vi "splice_intelligent_normalized_2.0.vi"(8 "xmax":dbl, 9 "xmin":dbl, 10 "X":dbl[](array[numeric]), 11 "Y":dbl[](array[numeric])) -> (0 "Splice indices":i32[](array[numeric]), 1 "Extrema type (T=max, F=min)":bool[](array[boolean]), 2 "X splices":cluster{dbl[]}[](array[cluster]), 3 "Y splices":cluster{dbl[]}[](array[cluster]), 4 "Extrema (indices)":i32[](array[numeric]))   [LabVIEW 2019]
uses:
  <vilib>/ptbypt/NI_PtbyPt.lvlib
panel:
  out "XY Graph":cluster{"X":dbl[], "Y":dbl[]}(graph)
  out "Array":cluster{"XY Graph":cluster{dbl[], dbl[]}}[](array[cluster])
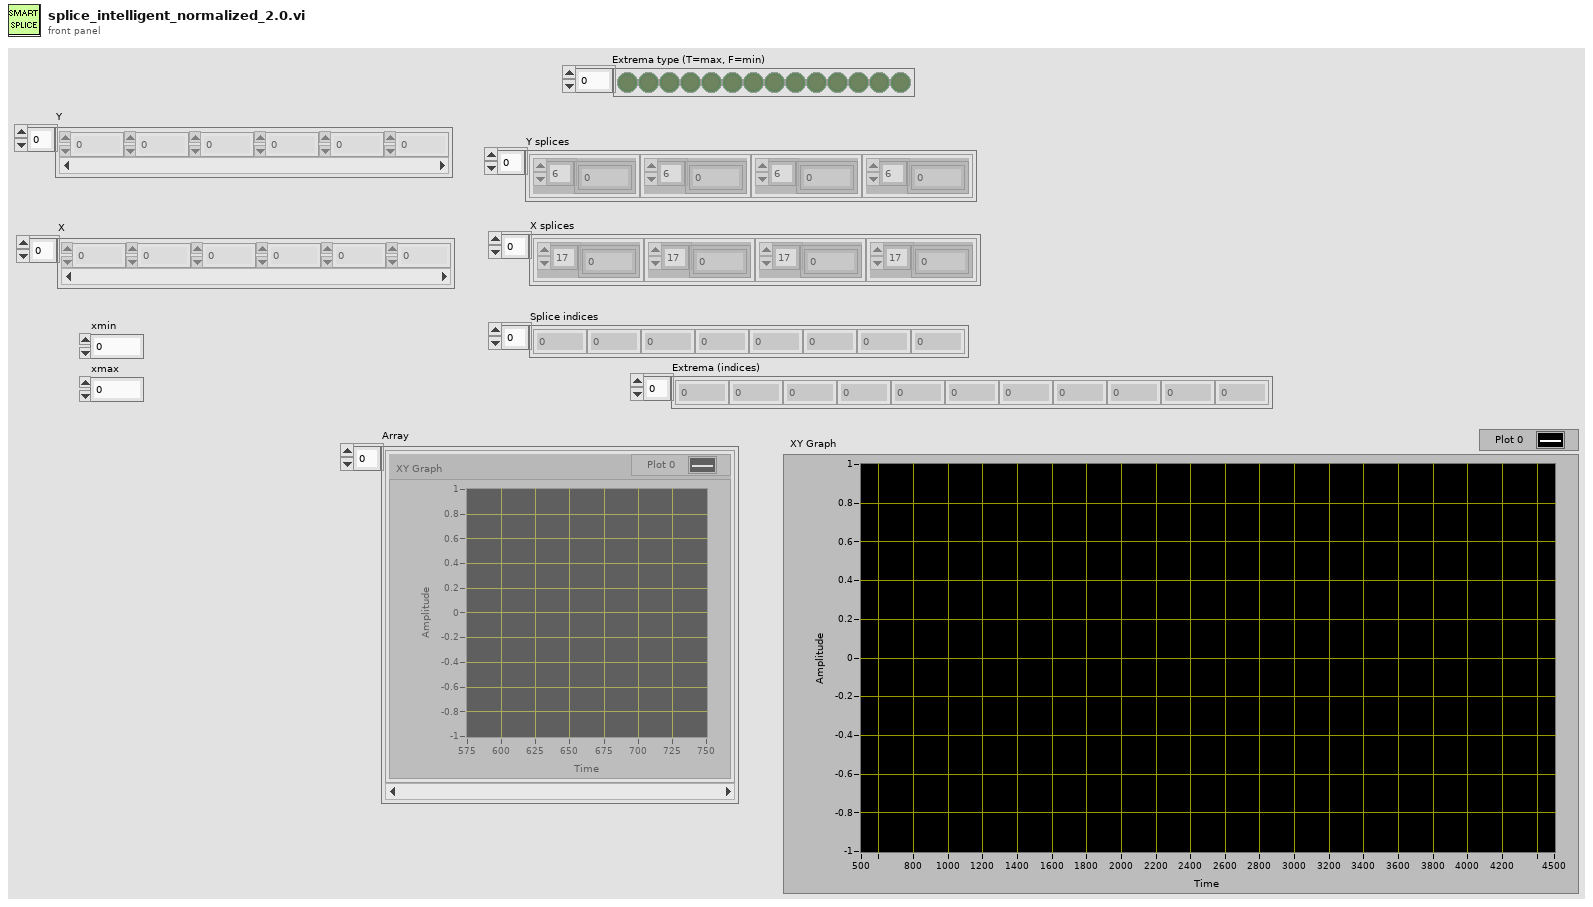
[diagram p1: front panel]
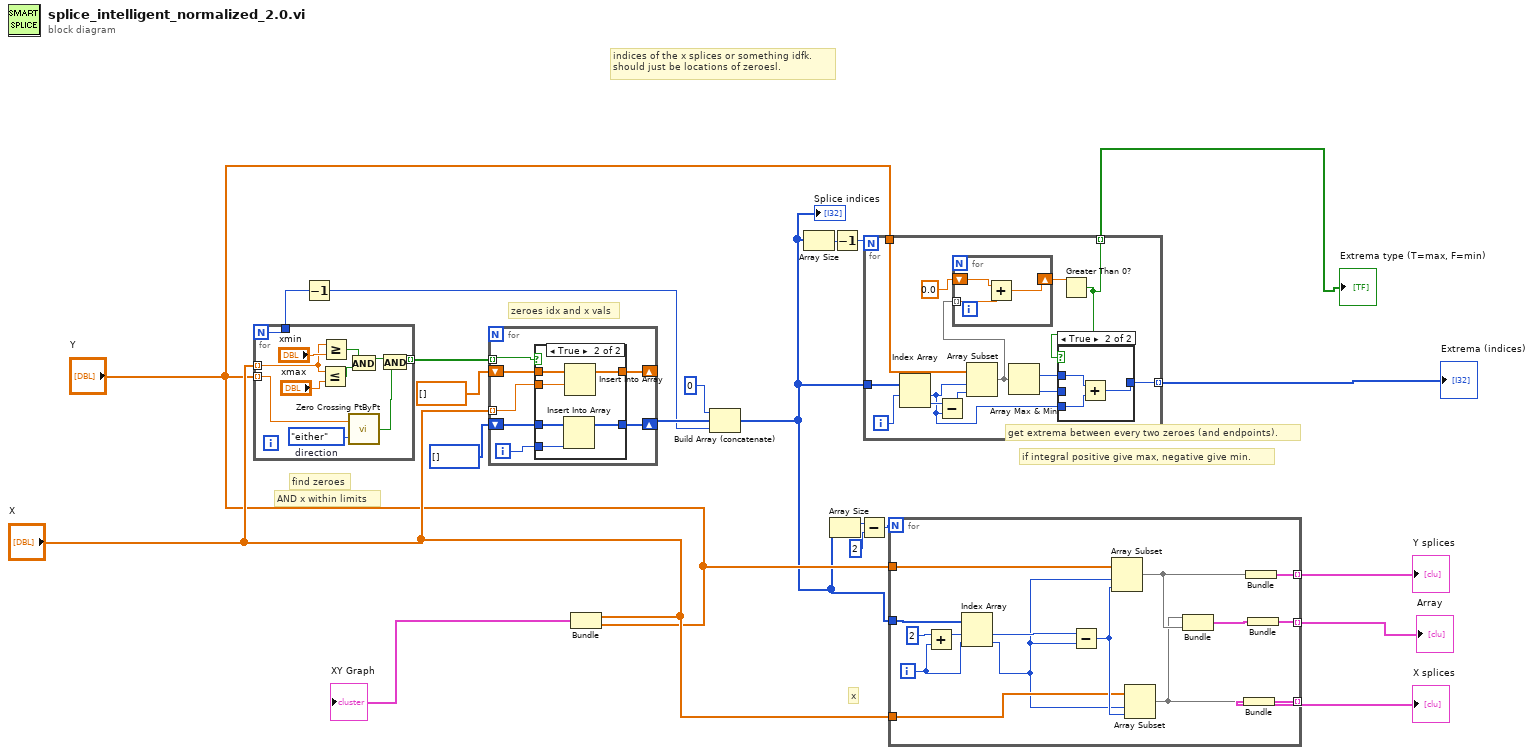
[diagram p0: block diagram]
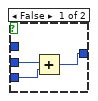
[diagram p2: hidden frame]
diagram:
  # "get extrema between every two zeroes (and endpoints)."
  # "zeroes idx and x vals"
  # "find zeroes"
  # "AND x within limits"
  # "indices of the x splices or something idfk. \nshould just be locations of zeroesl."
  # "if integral positive give max, negative give min."
  # "x"
  n1 = for {
    N -> [w22]
    tunnel: "Y" -> [w31] mode=indexing
    tunnel: [w25] -> w14 mode=indexing
    tunnel: "X" -> [w26] mode=indexing
    tunnel: [w22] -> w5
    w32 = enum16{"either", "minus-plus", "plus-minus"}."either"  # direction
    n2 = Less Or Equal?(x=w26, y="xmax") -> (x <= y?=w27:bool)
    n3 = Greater Or Equal?(x=w26, y="xmin") -> (x >= y?=w28:bool)
    n4 = And(x=w28, y=w27) -> (x .and. y?=w23:bool)
    n5 = call <vilib>:"Zero Crossing PtByPt.vi"("direction"=w32, "input data point"=w31) -> ("crossing"=w24:bool)  [unwired: 1 in]
    n6 = And(x=w23, y=w24) -> (x .and. y?=w25:bool)
  }
  n7 = Decrement(x=w5) -> (x-1=w4:i32)
  n8 = for {
    tunnel: "X" -> [w38] mode=indexing
    tunnel: w14 -> [w39] mode=indexing
    shift-right: [w36] -> _
    shift-left: dbl[] [] ("X") -> [w37]
    shift-right: [w33] -> w7
    shift-left: i32[] [] ("X") -> [w34]
    i -> [w35]
    n9 = case shown="True" w39 {
      tunnel: w38 -> [_ w46]
      tunnel: w37 -> [w41 w47]
      tunnel: [w41 w45] -> w36
      tunnel: w35 -> [_ w43]
      tunnel: w34 -> [w40 w44]
      tunnel: [w40 w42] -> w33
      frame False {
      }
      frame True {
        n10 = Insert Into Array(array=w44, new element=w43) -> (w42:i32[])  [unwired: 1 in]
        n11 = Insert Into Array(array=w47, new element=w46) -> (w45:dbl[])  [unwired: 1 in]
      }
    }
  }
  n12 = Bundle("X"="X", "Y"="Y") -> (→"XY Graph":cluster{"X":dbl[], "Y":dbl[]})  [unwired: 1 in]
  n13 = Build Array (concatenate)(0, w7, w4) -> (w2:i32[])
  "Splice indices" <- w2
  n14 = Array Size(array=w2) -> (size(s)=w10:i32)
  n15 = Array Size(array=w2) -> (size(s)=w19:i32)
  n16 = Decrement(x=w10) -> (x-1=w11:i32)
  n17 = Subtract(x=w19, y=2) -> (x-y=w18:i32)
  n18 = for {
    N: w11 -> [_]
    tunnel: [w50] -> w9 mode=indexing
    tunnel: "Y" -> [w60]
    tunnel: w2 -> [w59]
    tunnel: [w49] -> w1 mode=indexing
    i -> [w58]
    n19 = Index Array(array=w59, index #1=w58) -> (element #1=w48:i32, element #2=w57:i32)  [unwired: 1 in]
    n20 = Subtract(x=w57, y=w48) -> (x-y=w56:i32)
    n21 = Array Subset(array=w60, index=w48, length=w56) -> (w53:dbl[])
    n22 = for {
      tunnel: w53 -> [w62] mode=indexing
      shift-right: [w61] -> w54
      shift-left: 0.0 -> [w63]
      n23 = Add(x=w63, y=w62) -> (x+y=w61:dbl)
    }
    n24 = Array Max & Min(array=w53) -> (max index (indices)=w52:i32, min index (indices)=w51:i32)  [unwired: 2 out]
    n25 = Greater Than 0?(x=w54) -> (x > 0?=w49:bool)
    n26 = case shown="True" w49 {
      tunnel: w52 -> [_ w68]
      tunnel: w51 -> [w66 _]
      tunnel: [w64 w67] -> w50
      tunnel: w48 -> [w65 w69]
      frame False {
        n27 = Add(x=w66, y=w65) -> (x+y=w64:i32)
      }
      frame True {
        n28 = Add(x=w68, y=w69) -> (x+y=w67:i32)
      }
    }
  }
  "Extrema (indices)" <- w9
  "Extrema type (T=max, F=min)" <- w1
  n29 = for {
    N: w18 -> [_]
    tunnel: "Y" -> [w84]
    tunnel: [w81] -> w21 mode=indexing
    tunnel: w2 -> [w79]
    tunnel: "X" -> [w77]
    tunnel: [w76] -> w20 mode=indexing
    tunnel: [w72] -> w16 mode=indexing
    i -> [w71]
    n30 = Add(x=2, y=w71) -> (x+y=w83:i32)
    n31 = Index Array(array=w79, index #1=w83, index #2=w71) -> (element #1=w80:i32, element #2=w70:i32)
    n32 = Subtract(x=w80, y=w70) -> (x-y=w78:i32)
    n33 = Array Subset(array=w84, index=w70, length=w78) -> (w75:dbl[])
    n34 = Array Subset(array=w77, index=w70, length=w78) -> (w74:dbl[])
    n35 = Bundle(w74, w75) -> (w73:cluster{dbl[], dbl[]})  [unwired: 1 in]
    n36 = Bundle(w74) -> (w76:cluster{dbl[]})  [unwired: 1 in]
    n37 = Bundle(w75) -> (w81:cluster{dbl[]})  [unwired: 1 in]
    n38 = Bundle(w73) -> (w72:cluster{cluster{dbl[], dbl[]}})  [unwired: 1 in]
  }
  "Y splices" <- w21
  "X splices" <- w20
  "Array" <- w16
